vi "sbrio.vi"() -> ()   [LabVIEW 2012]
uses:
  <vilib>/rvi/interface/nirviOpenFPGA/nirviOpenFPGA.xnode
  <vilib>/rvi/interface/nirviMethod/nirviMethod.xnode
  <vilib>/FPGAPlugInAG/Dynamic/niLvFpga_Abort_Dynamic.vi
  <vilib>/FPGAPlugInAG/Dynamic/niLvFpga_Run_Dynamic.vi
  <vilib>/rvi/interface/nirviReadWriteControl/nirviReadWriteControl.xnode
  NiFpgaLv.dll
  <vilib>/Utility/error.llb/Error Cluster From Error Code.vi
  <vilib>/rvi/interface/Simulation/niFpgaSimulationCallBeginRW.vi
  <vilib>/rvi/errors/niLvFpgaAdjustHostInterfaceError.vi
  <vilib>/rvi/interface/nirviCloseFPGA/nirviCloseFPGA.xnode
  <vilib>/FPGAPlugInAG/Dynamic/niLvFpga_Close_Dynamic.vi
  <vilib>/NI_Real-Time Target Support.lvlib
  FPGA Bitfiles/autonomous_FPGATarget3_fpga_1WTnqbhggzA.lvbitx
  autocarnav4/RCcar/fpga.vi
  <vilib>/FPGAPlugInAG/sbRIO-9606/niLvFpga_Open_sbRIO-9606.vi
  <vilib>/rvi/interface/common/dynamic/niFpgaDynamicAddResources.vi
panel:
  in  "Double":dbl
  out "steer_input":dbl
  out "FPGA":refnum<k20>
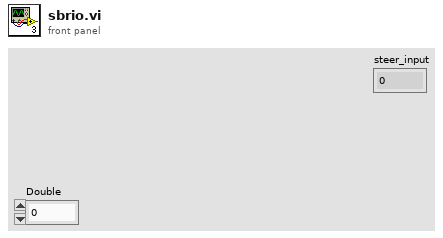
[diagram p1: front panel]
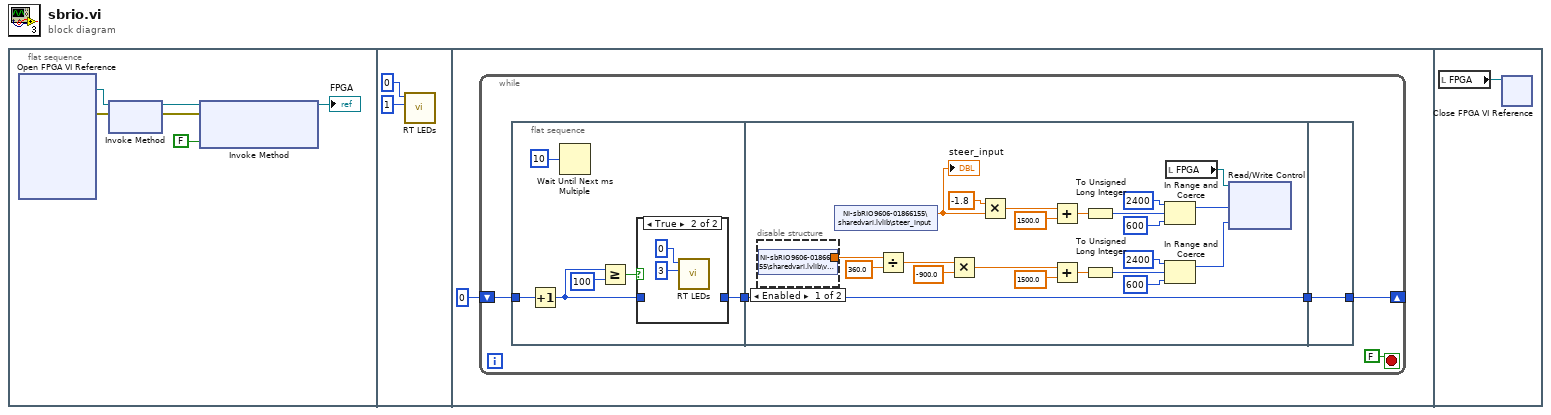
[diagram p0: block diagram]
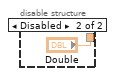
[diagram p3: hidden frame]
diagram:
  n1 = flat-sequence {
    frame #0 {
      n2 = xnode "Open FPGA VI Reference"() -> ("FPGA VI Reference Out"=w6:refnum<k20>, "error out"=w5:errorcluster)  [unwired: 2 in]
      n3 = xnode "Invoke Method"("FPGA VI Reference In"=w6, "error in"=w5) -> ("FPGA VI Reference Out"=w4:refnum<k20>, "error out"=w3:errorcluster)
      n4 = xnode "Invoke Method"("FPGA VI Reference In"=w4, "error in"=w3, "Wait Until Done (F)"=FALSE) -> ("FPGA VI Reference Out"=→"FPGA":refnum<k20>)  [unwired: 1 out]
    }
    frame #1 {
      n5 = call <vilib>:"RT LEDs.vi"("State"=1, "LED Num"=0) -> ()  [unwired: 4 in, 2 out]
    }
    frame #2 {
      n6 = while {
        shift-right: [w12] -> _
        shift-left: u32 0 ("millisecond multiple") -> [w13]
        stop <- FALSE stop-if-true
        n7 = flat-sequence {
          tunnel: w13 -> [w19]
          tunnel: [w15] -> w10
          tunnel: [w24] -> w11
          tunnel: w10 -> [w24]
          tunnel: [w48] -> w12
          tunnel: w11 -> [w48]
          frame #0 {
            n8 = Increment(x=w19) -> (x+1=w16:u32)
            n9 = Wait Until Next ms Multiple(millisecond multiple=u32 10) -> ()  [unwired: 1 out]
            n10 = Greater Or Equal?(x=w16, y=u32 100) -> (x >= y?=w17:bool)
            n11 = case shown="True" w17 {
              tunnel: w16 -> [w21 _]
              tunnel: [w21 _] -> w15
              frame False {
              }
              frame True {
                n12 = call <vilib>:"RT LEDs.vi"("State"=3, "LED Num"=0) -> ()  [unwired: 4 in, 2 out]
              }
            }
          }
          frame #1 {
            n13 = disable-structure shown="Enabled" {
              disable-tunnel: [w46 "Double"] -> w35
              frame Enabled {
                n14 = shared-variable "NI-sbRIO9606-01866155\\sharedvari.lvlib\\vs_des"() -> (w46:dbl)  [unwired: 1 in, 1 out]
              }
              frame Disabled {
              }
            }
            n15 = shared-variable "NI-sbRIO9606-01866155\\sharedvari.lvlib\\steer_input"() -> (w43:dbl)  [unwired: 1 in, 1 out]
            "steer_input" <- w43
            n16 = Divide(x=w35, y=360.0) -> (x/y=w33:dbl)
            n17 = Multiply(x=w33, y=-900.0) -> (x*y=w30:dbl)
            n18 = Multiply(x=-1.8, y=w43) -> (x*y=w42:dbl)
            n19 = Add(x=w42, y=1500.0) -> (x+y=w40:dbl)
            n20 = Add(x=w30, y=1500.0) -> (x+y=w26:dbl)
            n21 = To Unsigned Long Integer(number=w40) -> (unsigned 32bit integer=w39:u32)
            n22 = To Unsigned Long Integer(number=w26) -> (unsigned 32bit integer=w27:u32)
            n23 = In Range and Coerce(upper limit=u32 2400, x=w39, lower limit=u32 600) -> (coerced(x)=w36:u32)  [unwired: 1 out]
            n24 = In Range and Coerce(upper limit=u32 2400, x=w27, lower limit=u32 600) -> (coerced(x)=w25:u32)  [unwired: 1 out]
            n25 = local read "FPGA"() -> (w45:refnum<k20>)
            n26 = xnode "Read/Write Control"("FPGA VI Reference In"=w45, "PWM 15"=w36, "PWM 31"=w25) -> ()  [unwired: 1 in, 2 out]
          }
          frame #2 {
          }
        }
      }
    }
    frame #3 {
      n27 = local read "FPGA"() -> (w49:refnum<k20>)
      n28 = xnode "Close FPGA VI Reference"("FPGA VI Reference In"=w49) -> ()  [unwired: 1 in, 1 out]
    }
  }
